vi "Chang all cell colors.vi"(6 "F： Clear Table Data":bool, 7 "ColumnNum":i32, 8 "error in (no error)":errorcluster, 9 "Color Box":u32(colorbox)=16448250, 10 "Row Num":i32=50, 11 "Multicolumn Listbox In":refnum<vi>) -> (0 "error out":errorcluster, 3 "Multicolumn Listbox Out":refnum<vi>)   [LabVIEW 2021]
uses:
  <vilib>/Utility/miscctls.llb/LVRowAndColumnTypeDef.ctl
  <vilib>/Utility/miscctls.llb/LVRowAndColumnUnsignedTypeDef.ctl
panel:
  in  "s":bool
  in  "Multicolumn Listbox":i32[](listbox)
  out "size(s)":i32[](array[numeric])
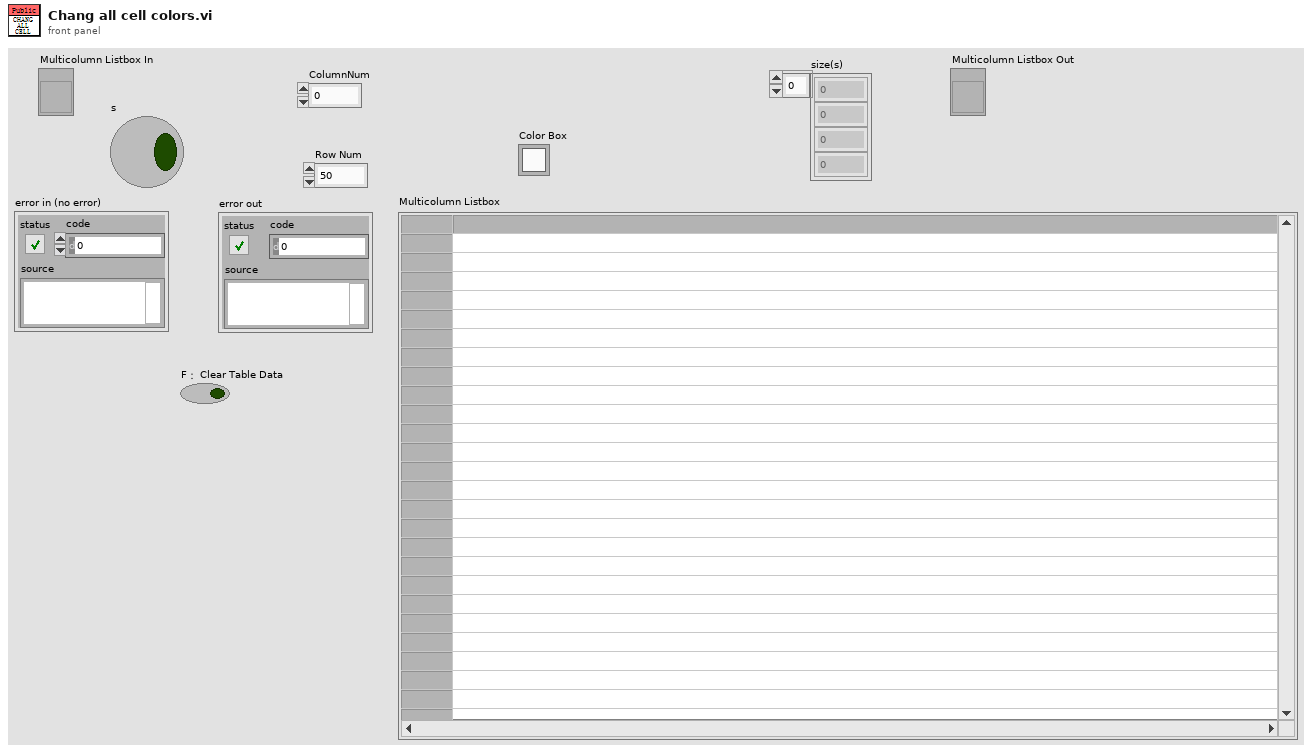
[diagram p1: front panel]
types:
  T1 = typedef "LVRowAndColumnTypeDef.ctl" = cluster{"Row":i32, "Column":i32}
  T2 = typedef "LVRowAndColumnUnsignedTypeDef.ctl" = cluster{"Row":u32, "Column":u32}
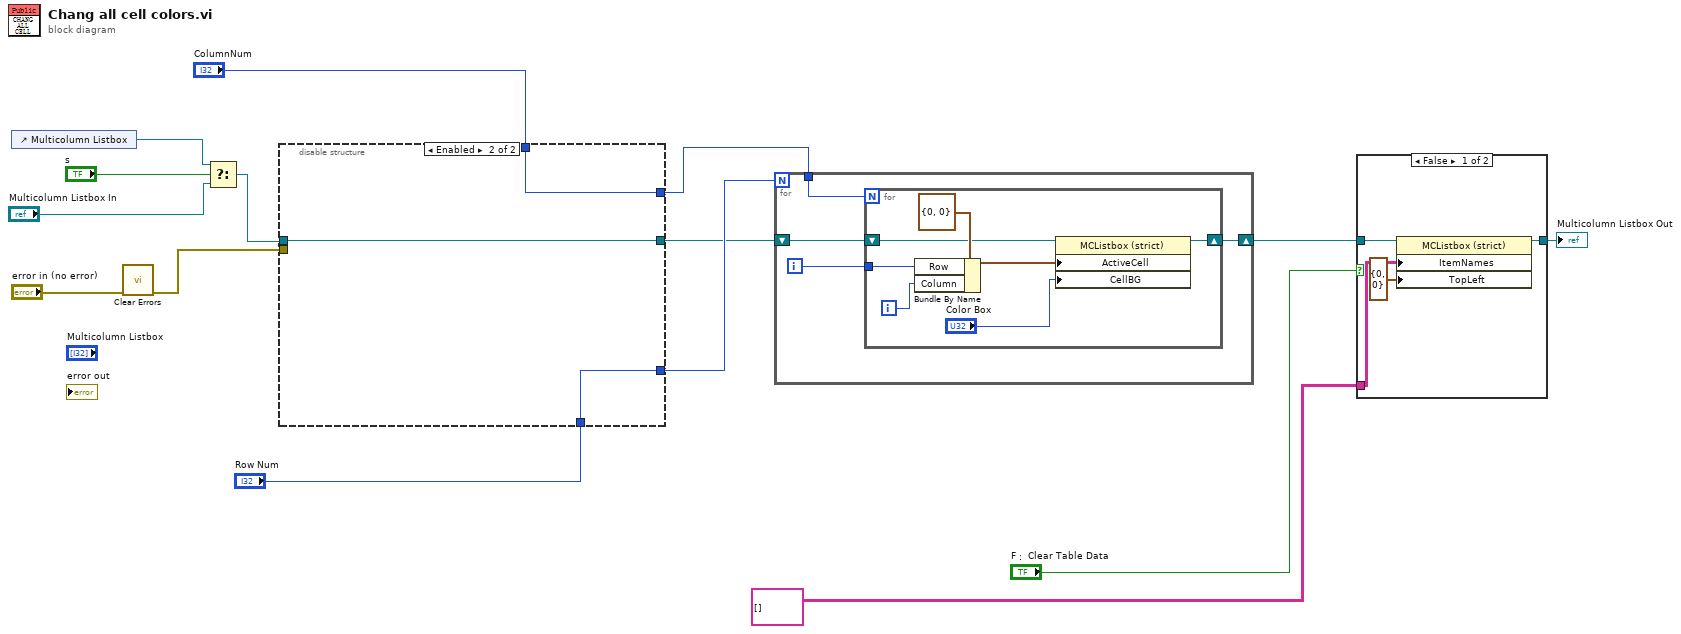
[diagram p0: block diagram]
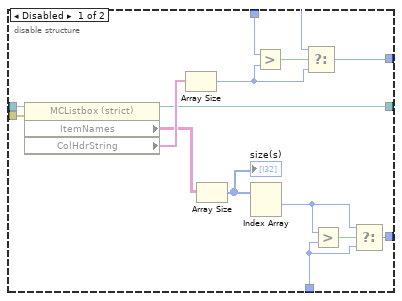
[diagram p2: hidden frame]
diagram:
  n1 = control-ref of="Multicolumn Listbox"() -> (w3:refnum<vi>)
  n2 = call <vilib>:"Clear Errors.vi"("error in (no error)"="error in (no error)") -> ("error out"=w4:errorcluster)  [unwired: 5 in, 1 out]
  n3 = Select(t=w3, s="s", f="Multicolumn Listbox In") -> (s? t:f=w1:refnum<vi>)
  n4 = disable-structure shown="Enabled" {
    disable-tunnel: [w29 w32] -> w12
    disable-tunnel: "ColumnNum" -> [w27 w32]
    disable-tunnel: [w25 w30] -> w10
    disable-tunnel: "Row Num" -> [w23 w30]
    disable-tunnel: [w20 w31] -> w6
    disable-tunnel: w4 -> [w19 _]
    disable-tunnel: w1 -> [w18 w31]
    frame Disabled {
      n5 = property class="MCListbox (strict)"(reference=w18, error in=w19) -> (reference out=w20:refnum<vi>, "ItemNames"=w17:string[][], "ColHdrString"=w21:string[])  [unwired: 1 out]
      n6 = Array Size(array=w21) -> (size(s)=w28:i32)
      n7 = Array Size(array=w17) -> (size(s)=w16:i32[])
      "size(s)" <- w16
      n8 = Index Array(array=w16) -> (element #1=w24:i32)  [unwired: 2 in, 1 out]
      n9 = Greater?(x=w27, y=w28) -> (0:w26:bool)
      n10 = Select(t=w27, s=w26, f=w28) -> (s? t:f=w29:i32)
      n11 = Greater?(x=w24, y=w23) -> (0:w22:bool)
      n12 = Select(t=w24, s=w22, f=w23) -> (s? t:f=w25:i32)
    }
    frame Enabled {
    }
  }
  n13 = for {
    N: w10 -> [_]
    tunnel: w12 -> [w35]
    shift-right: [w33] -> w7
    shift-left: w6 -> [w34]
    i -> [w36]
    n14 = for {
      N: w35 -> [_]
      tunnel: w36 -> [w40]
      shift-right: [w38] -> w33
      shift-left: w34 -> [w39]
      i -> [w41]
      n15 = Bundle By Name(cluster=T1 {"Row"=0, "Column"=0} ("Active Cell:Active Cell"), "Row"=w40, "Column"=w41) -> (w42:T1)
      n16 = property on="Property Node" class="MCListbox (strict)"(reference=w39, "ActiveCell"=w42, "CellBG"="Color Box") -> (reference out=w38:refnum<vi>)  [unwired: 1 in, 1 out]
    }
  }
  n17 = case shown="False" "F： Clear Table Data" {
    tunnel: w7 -> [w47 w48]
    tunnel: [w46 w48] -> w15
    tunnel: string[][] [] ("Item Names") -> [w45 _]
    frame False {
      n18 = property class="MCListbox (strict)"(reference=w47, "ItemNames"=w45, "TopLeft"=T2 {"Row"=0, "Column"=0} ("Top Left Visible Cell")) -> (reference out=w46:refnum<vi>)  [unwired: 1 in, 1 out]
    }
    frame True {
    }
  }
  "Multicolumn Listbox Out" <- w15
